vi "Teleop Climb Control.vi"(11 "Button Cluster":T1) -> ()   [LabVIEW 2016]
uses:
  Common Code/Gamepads/Button Cluster.ctl
  Robot Global Data.vi
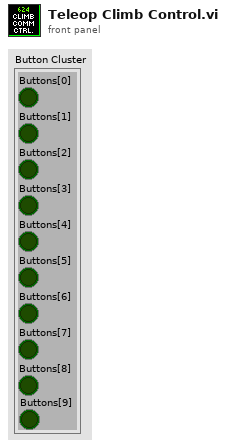
[diagram p1: front panel]
types:
  T1 = typedef "Button Cluster.ctl" = cluster{"Buttons[0]":bool, "Buttons[1]":bool, "Buttons[2]":bool, "Buttons[3]":bool, "Buttons[4]":bool, "Buttons[5]":bool, "Buttons[6]":bool, "Buttons[7]":bool, "Buttons[8]":bool, "Buttons[9]":bool}
  T2 = typedef "Climb Command Cluster.ctl" = cluster{"Go Up":bool, "Go Down":bool}
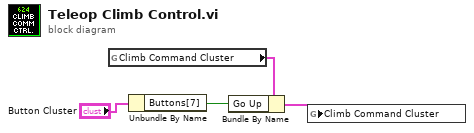
[diagram p0: block diagram]
diagram:
  n1 = global read "Robot Global Data.vi" "Climb Command Cluster"() -> (w3:T2)
  n2 = Unbundle By Name("Button Cluster") -> ("Buttons[7]"=w1:bool)
  n3 = Bundle By Name(cluster=w3, "Go Up"=w1) -> (w2:T2)
  n4 = global write "Robot Global Data.vi" "Climb Command Cluster"(w2) -> ()
